vi "mso7014b_init.vi"(8 "Trigger Source (0: Channel 1)":u16(ring) items=["Channel 1", "Channel 2", "Channel 3", "Channel 4", "DIG 0", "DIG 1", "DIG 2", "DIG 3", "DIG 4", "DIG 5", "DIG 6", "DIG 7", "DIG 8", "DIG 9", "DIG 10", "DIG 11", "DIG 12", "DIG 13", "DIG 14", "DIG 15", "Line", "External"], 9 "Trigger Level (V)":dbl=0.3 format="%#_13g", 10 "Oscilloscope IO":refnum<visa-resource-name>="tcpip0::192.168.40.70::instr", 11 "Timebase (20.0E-9)":dbl=0.004 format="%#_13g") -> (0 "dt":dbl, 1 "error out":errorcluster, 2 "VISA resource name out":refnum<visa-resource-name>)   [LabVIEW 2016]
uses:
  <instrlib>/Agilent 6000 Series/Public/Configure/Configure Edge Trigger Source.vi
  <instrlib>/Agilent 6000 Series/Agilent 6000 Series.lvlib
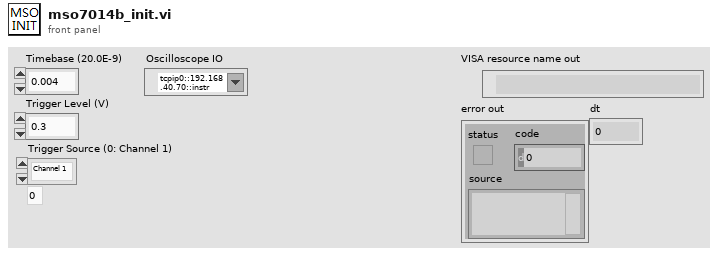
[diagram p1: front panel]
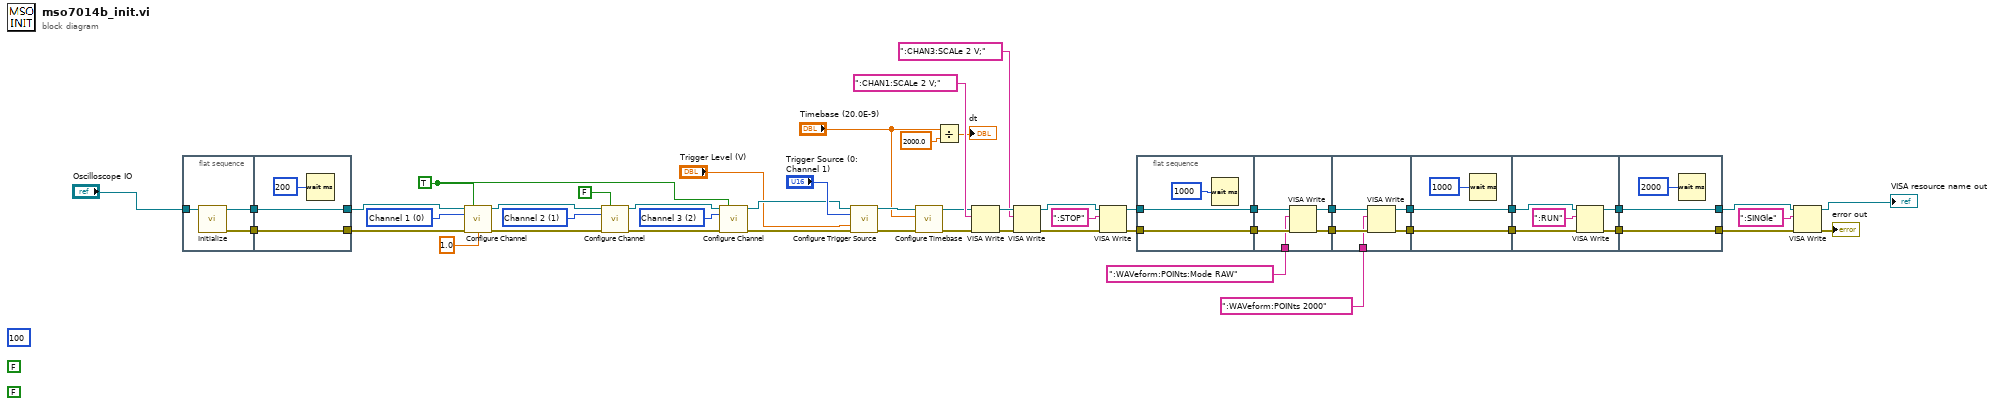
[diagram p0: block diagram]
diagram:
  (unwired) FALSE ("Continuous Acquisition Mode (T: Enable)")
  (unwired) FALSE ("Continuous Acquisition Mode (T: Enable)")
  (unwired) u32 100 ("字节总数")
  w35 = u16 0 items=["Channel 1", "Channel 2", "Channel 3", "Channel 4"] ("Channel (0: Channel 1)")
  w44 = TRUE ("Enable Channel (T: Enable)")
  w47 = u16 2 items=["Channel 1", "Channel 2", "Channel 3", "Channel 4"] ("Channel (0: Channel 1)")
  w49 = u16 1 items=["Channel 1", "Channel 2", "Channel 3", "Channel 4"] ("Channel (0: Channel 1)")
  n1 = flat-sequence {
    tunnel: "Oscilloscope IO" -> [w55]
    tunnel: [w54] -> w9
    tunnel: [w53] -> w8
    tunnel: [w57] -> w41
    tunnel: [w58] -> w42
    tunnel: w9 -> [w58]
    tunnel: w8 -> [w57]
    frame #0 {
      n2 = call <instrlib>:"Initialize.vi"("VISA resource name"=w55) -> ("error out"=w53:errorcluster, "VISA resource name out"=w54:refnum<visa-resource-name>)  [unwired: 9 in]
    }
    frame #1 {
      n3 = Wait (ms)(milliseconds to wait=u32 200 ("等待时间（毫秒）")) -> ()  [unwired: 1 out]
    }
  }
  n4 = call <instrlib>:"Configure Channel.vi"("VISA resource name"=w42, "Enable Channel (T: Enable)"=w44, "Channel (0: Channel 1)"=w35, "error in (no error)"=w41, "Vertical Offset (0.0 V)"=1.0) -> ("VISA resource name out"=w51:refnum<visa-resource-name>, "error out"=w46:errorcluster)  [unwired: 9 in]
  n5 = call <instrlib>:"Configure Channel.vi"("VISA resource name"=w51, "Enable Channel (T: Enable)"=FALSE, "Channel (0: Channel 1)"=w49, "error in (no error)"=w46) -> ("VISA resource name out"=w50:refnum<visa-resource-name>, "error out"=w45:errorcluster)  [unwired: 10 in]
  n6 = call <instrlib>:"Configure Channel.vi"("VISA resource name"=w50, "Enable Channel (T: Enable)"=w44, "Channel (0: Channel 1)"=w47, "error in (no error)"=w45) -> ("VISA resource name out"=w40:refnum<visa-resource-name>, "error out"=w39:errorcluster)  [unwired: 10 in]
  n7 = call-poly <instrlib>:"Configure Trigger Source.vi"("VISA resource name"=w40, "Trigger Source (0: Channel 1)"="Trigger Source (0: Channel 1)", "Trigger Level (0.0 V)"="Trigger Level (V)", "error in (no error)"=w39) -> ("VISA resource name out"=w38:refnum<visa-resource-name>, "error out"=w37:errorcluster)  [unwired: 10 in]
  n8 = call <instrlib>:"Configure Timebase.vi"("error in (no error)"=w37, "Timebase (20.0E-9)"="Timebase (20.0E-9)", "VISA resource name"=w38) -> ("error out"=w31:errorcluster, "VISA resource name out"=w32:refnum<visa-resource-name>)  [unwired: 7 in]
  n9 = Divide(x="Timebase (20.0E-9)", y=2000.0) -> (x/y=→"dt":dbl)
  n10 = VISA Write(VISA resource name=w32, write buffer=":CHAN1:SCALe 2 V;" ("写入缓冲区"), error in (no error)=w31) -> (VISA resource name out=w5:refnum<visa-resource-name>, error out=w4:errorcluster)  [unwired: 1 out]
  n11 = VISA Write(VISA resource name=w5, write buffer=":CHAN3:SCALe 2 V;" ("写入缓冲区"), error in (no error)=w4) -> (VISA resource name out=w3:refnum<visa-resource-name>, error out=w2:errorcluster)  [unwired: 1 out]
  n12 = VISA Write(VISA resource name=w3, write buffer=":STOP" ("写入缓冲区"), error in (no error)=w2) -> (VISA resource name out=w27:refnum<visa-resource-name>, error out=w26:errorcluster)  [unwired: 1 out]
  n13 = flat-sequence {
    tunnel: w27 -> [w61]
    tunnel: w26 -> [w60]
    tunnel: [w61] -> w22
    tunnel: [w60] -> w21
    tunnel: w22 -> [w66]
    tunnel: w21 -> [w65]
    tunnel: [w64] -> w20
    tunnel: [w63] -> w19
    tunnel: ":WAVeform:POINts:Mode RAW" ("写入缓冲区") -> [w62]
    tunnel: w20 -> [w71]
    tunnel: w19 -> [w70]
    tunnel: ":WAVeform:POINts 2000" ("写入缓冲区") -> [w69]
    tunnel: [w68] -> w15
    tunnel: [w67] -> w13
    tunnel: w15 -> [w74]
    tunnel: [w74] -> w14
    tunnel: w13 -> [w73]
    tunnel: [w73] -> w12
    tunnel: w14 -> [w79]
    tunnel: w12 -> [w78]
    tunnel: [w77] -> w11
    tunnel: [w76] -> w10
    tunnel: [w81] -> w28
    tunnel: [w82] -> w29
    tunnel: w11 -> [w82]
    tunnel: w10 -> [w81]
    frame #0 {
      n14 = Wait (ms)(milliseconds to wait=u32 1000 ("等待时间（毫秒）")) -> ()  [unwired: 1 out]
    }
    frame #1 {
      n15 = VISA Write(VISA resource name=w66, write buffer=w62, error in (no error)=w65) -> (VISA resource name out=w64:refnum<visa-resource-name>, error out=w63:errorcluster)  [unwired: 1 out]
    }
    frame #2 {
      n16 = VISA Write(VISA resource name=w71, write buffer=w69, error in (no error)=w70) -> (VISA resource name out=w68:refnum<visa-resource-name>, error out=w67:errorcluster)  [unwired: 1 out]
    }
    frame #3 {
      n17 = Wait (ms)(milliseconds to wait=u32 1000 ("等待时间（毫秒）")) -> ()  [unwired: 1 out]
    }
    frame #4 {
      n18 = VISA Write(VISA resource name=w79, write buffer=":RUN" ("写入缓冲区"), error in (no error)=w78) -> (VISA resource name out=w77:refnum<visa-resource-name>, error out=w76:errorcluster)  [unwired: 1 out]
    }
    frame #5 {
      n19 = Wait (ms)(milliseconds to wait=u32 2000 ("等待时间（毫秒）")) -> ()  [unwired: 1 out]
    }
  }
  n20 = VISA Write(VISA resource name=w29, write buffer=":SINGle" ("写入缓冲区"), error in (no error)=w28) -> (VISA resource name out=→"VISA resource name out":refnum<visa-resource-name>, error out=→"error out":errorcluster)  [unwired: 1 out]
